vi "Report.vi"(6 "Prompt to add new approved file to project? (T)":bool=TRUE, 8 "error in":errorcluster, 9 "Received":path, 10 "Approved":path, 11 "Reporter in":refnum<class "Reporter.lvclass">) -> (0 "error out":errorcluster, 2 "Worked?":bool, 3 "Reporter out":refnum<class "Reporter.lvclass">)   [LabVIEW 2020, in "Approval Tests.lvlib" / "Reporter.lvclass"]
uses:
  Reporter.lvclass
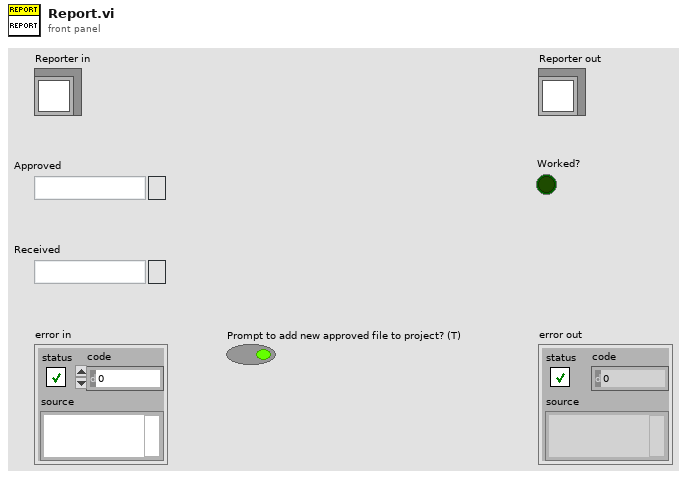
[diagram p1: front panel]
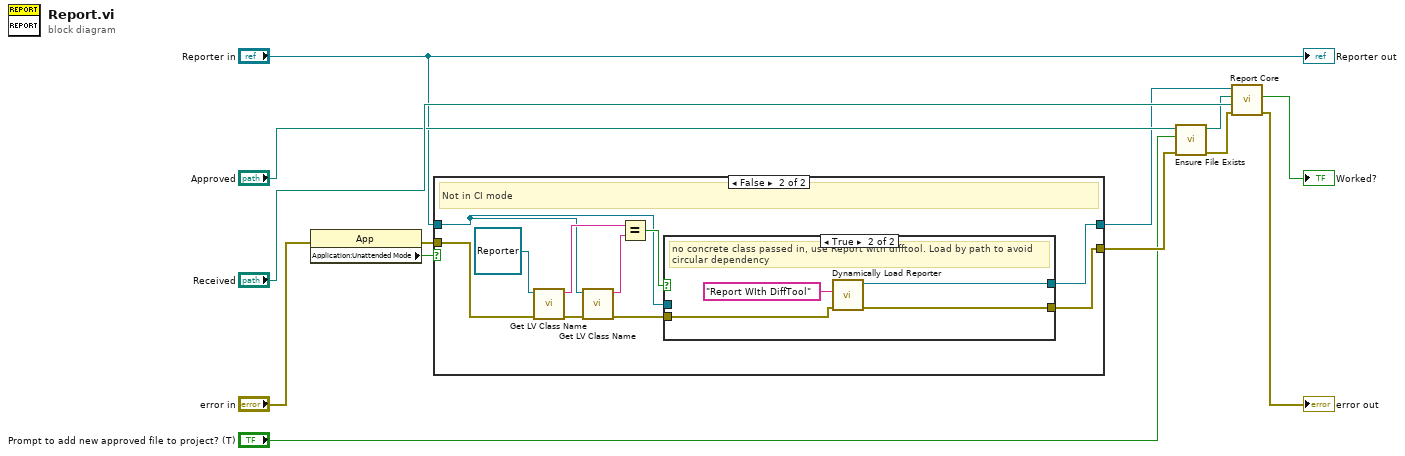
[diagram p0: block diagram]
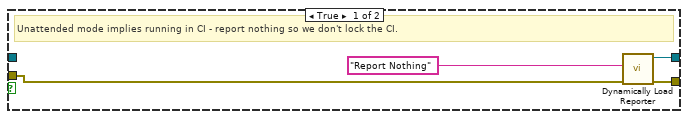
[diagram p2: hidden frame]
diagram:
  n1 = property class="App"(error in="error in") -> (error out=w9:errorcluster, "Application:Unattended Mode"=w1:bool)  [unwired: 1 in, 1 out]
  n2 = case shown="False" w1 {
    tunnel: "Reporter in" -> [_ w20]
    tunnel: [w14 w19] -> w3
    tunnel: [w16 w27] -> w11
    tunnel: w9 -> [w17 w26]
    frame True {
      # "Unattended mode implies running in CI - report nothing so we don't lock the CI."
      n3 = call "Dynamically Load Reporter.vi"("error in"=w17, "Reporter without ext"="Report Nothing") -> ("error out"=w16:errorcluster, "Approval Tests:Reporter"=w14:refnum<class "Reporter.lvclass">)  [unwired: 8 in]
    }
    frame False {
      # "Not in CI mode"
      n4 = call <vilib>:"Get LV Class Name.vi"("error in (no error)"=w26, "object"=refnum<class "Reporter.lvclass"> refnum ("Reporter in")) -> ("error out"=w25:errorcluster, "class name"=w23:string)  [unwired: 8 in]
      n5 = call <vilib>:"Get LV Class Name.vi"("error in (no error)"=w25, "object"=w20) -> ("error out"=w24:errorcluster, "class name"=w22:string)  [unwired: 8 in]
      n6 = Equal?(x=w23, y=w22) -> (x = y?=w21:bool)
      n7 = case shown="True" w21 {
        tunnel: w20 -> [w28 _]
        tunnel: [w28 w30] -> w19
        tunnel: [w29 w32] -> w27
        tunnel: w24 -> [w29 w33]
        frame False {
          # "some concrete object passed in - use that."
        }
        frame True {
          # "no concrete class passed in, use Report with difftool. Load by path to avoid circular dependency"
          n8 = call "Dynamically Load Reporter.vi"("error in"=w33, "Reporter without ext"="Report WIth DiffTool") -> ("error out"=w32:errorcluster, "Approval Tests:Reporter"=w30:refnum<class "Reporter.lvclass">)  [unwired: 8 in]
        }
      }
    }
  }
  n9 = call "Ensure File Exists.vi"("error in"=w11, "Prompt to add new approved file to project?"="Prompt to add new approved file to project? (T)", "Approved"="Approved") -> ("error out"=w12:errorcluster, "File Path"=w5:path)  [unwired: 7 in]
  n10 = call-dynamic "Report Core.vi"("error in"=w12, "Received"="Received", "Approved"=w5, "Reporter in"=w3) -> ("error out"=→"error out":errorcluster, "Worked?"=→"Worked?":bool)  [unwired: 5 in, 1 out]
  "Reporter out" <- "Reporter in"
